vi "RT Initialize Input Image (SubVI).vi"(8 "error in (no error)":errorcluster, 10 "Image Type":T2 items=["Grayscale (U8)", "Grayscale (I16)", "Grayscale (SGL)", "Complex (CSG)", "RGB (U32)", "HSL (U32)", "RGB (U64)", "Grayscale (U16)"], 11 "Image Size In":T1) -> (0 "error out":errorcluster, 2 "Input Image Size Out":T1, 3 "Input Image Out":T3)   [LabVIEW 2025, in "SoC IP Library.lvlib"]
uses:
  SoC IP Library.lvlib
  Controls/Image Size.ctl
  <vilib>/vision/Image Controls.llb/IMAQ Image.ctl
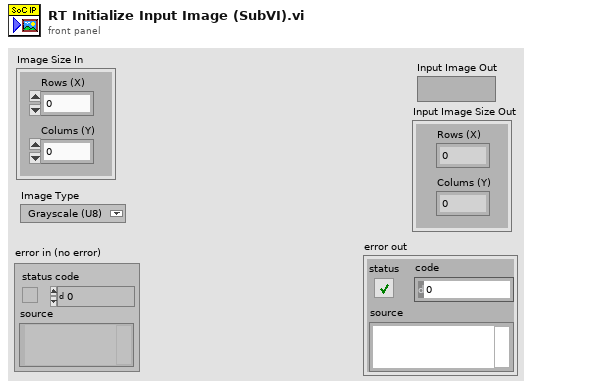
[diagram p1: front panel]
types:
  T1 = typedef "SoC IP Library.lvlib/Image Size.ctl" = cluster{"Rows (X)":u16, "Colums (Y)":u16}
  T2 = typedef "Image Type" = u32
  T3 = typedef "IMAQ Image.ctl" = refnum<image>
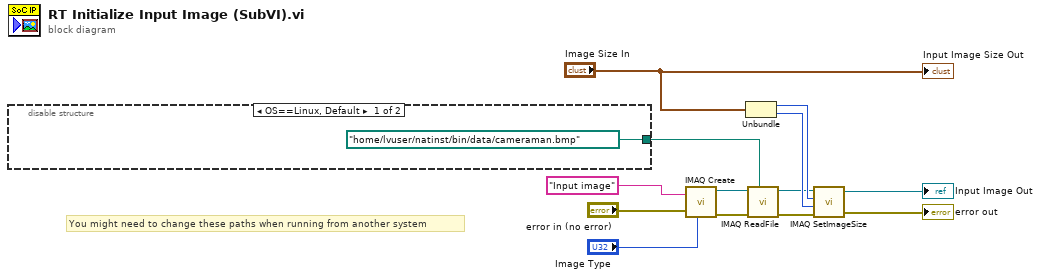
[diagram p0: block diagram]
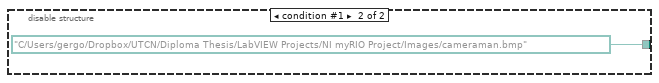
[diagram p2: hidden frame]
diagram:
  # "You might need to change these paths when running from another system"
  n1 = disable-structure shown="OS==Linux, Default" {
    disable-tunnel: [path "/home/lvuser/natinst/bin/data/cameraman.bmp" ("File Path") path "C:/Users/gergo/Dropbox/UTCN/Diploma Thesis/LabVIEW Projects/NI myRIO Project/Images/cameraman.bmp" ("File Path")] -> w5
    frame condition #0 (active) {
    }
    frame condition #1 {
    }
  }
  n2 = call "IMAQ Create"("Image Name"="Input image", "Image Type"="Image Type", "error in (no error)"="error in (no error)") -> ("New Image"=w8:T3, "error out"=w7:errorcluster)  [unwired: 2 in]
  n3 = Unbundle("Image Size In") -> ("Rows (X)"=w3:u16, "Colums (Y)"=w4:u16)
  n4 = call "IMAQ ReadFile"("File Path"=w5, "error in (no error)"=w7, "Image"=w8) -> ("error out"=w1:errorcluster, "Image Out"=w2:T3)  [unwired: 4 in, 3 out]
  n5 = call "IMAQ SetImageSize"("error in (no error)"=w1, "Y Resolution"=w4, "X Resolution"=w3, "Image"=w2) -> ("error out"=→"error out":errorcluster, "Image Out"=→"Input Image Out":T3)  [unwired: 1 in]
  "Input Image Size Out" <- "Image Size In"
